vi "Close Last File.vi"(8 "error in (no error)":errorcluster, 11 "[M] TDMS Save in":refnum<class "[M] TDMS Save.lvclass">) -> (0 "error out":errorcluster, 3 "[M] TDMS Save out":refnum<class "[M] TDMS Save.lvclass">)   [LabVIEW 2020, in "[M] TDMS Save.lvlib" / "[M] TDMS Save.lvclass"]
uses:
  [M] TDMS Save.lvclass
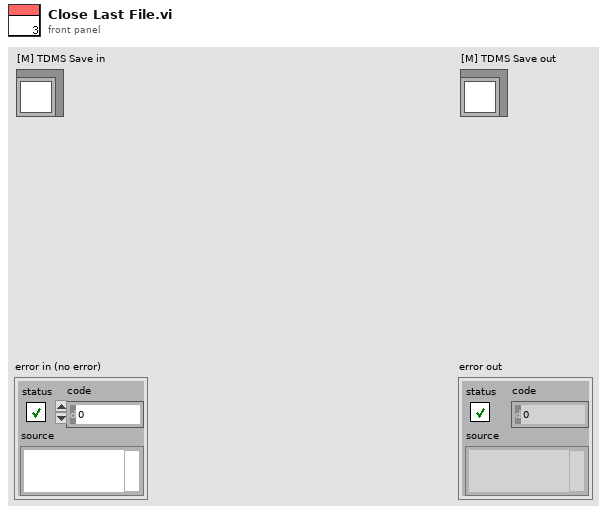
[diagram p1: front panel]
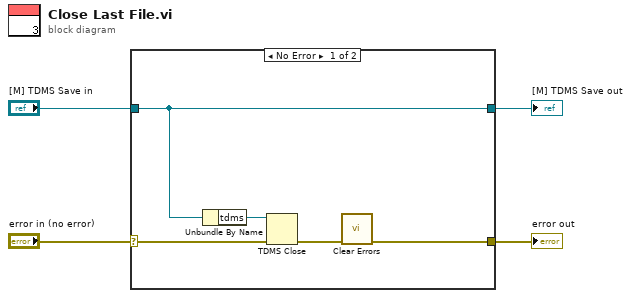
[diagram p0: block diagram]
diagram:
  n1 = case shown="No Error" "error in (no error)" {
    selector: "error in (no error)" -> [w8 w11]
    tunnel: [w5 w11] -> w3
    tunnel: [w9 w10] -> w1
    tunnel: "[M] TDMS Save in" -> [w9 w10]
    frame No Error {
      n2 = Unbundle By Name(w9) -> ("tdms"=w7:refnum<k34>)
      n3 = TDMS Close(8:w8, 11:w7) -> (0:w6:errorcluster)  [unwired: 1 out]
      n4 = call <vilib>:"Clear Errors.vi"("error in (no error)"=w6) -> ("error out"=w5:errorcluster)  [unwired: 5 in, 1 out]
    }
    frame Error {
    }
  }
  "error out" <- w3
  "[M] TDMS Save out" <- w1
